vi "_emi_Version from VI tags.vi"(0 "vi reference":refnum<vi>, 11 "error in":errorcluster) -> (4 "vi Refnum out":refnum<vi>, 8 "Version Info":T1 {"Date" format="%<%y%m%d>T"}, 15 "error out":errorcluster)   [LabVIEW 2010]
doc: "Reads version information from a VI.\n\nIf it fails it does not transmitt error information on."
uses:
  emi_Version Info.ctl
  <vilib>/UserTags/UserTags.lvlib
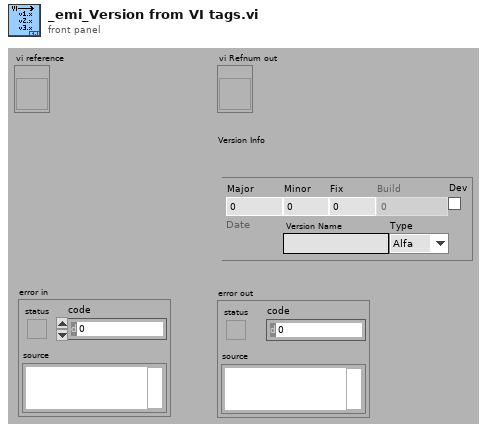
[diagram p1: front panel]
types:
  T1 = typedef "emi_Version Info.ctl" = cluster{"Name":string, "Major":i16, "Minor":i16, "Fix":i16, "Build":i32, "Type":enum16{"Alfa", "Beta", "Stable"}, "Dev":bool, "Version Name":string, "Date":timestamp}
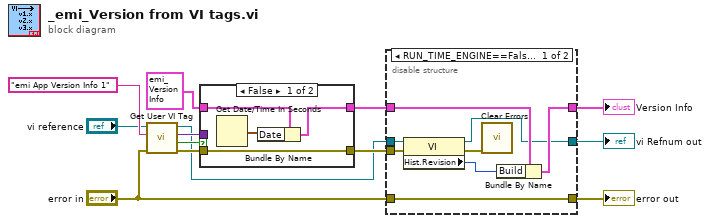
[diagram p0: block diagram]
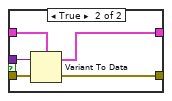
[diagram p3: hidden frame]
diagram:
  n1 = call <vilib>:"Get User VI Tag.vi"("error in (no error)"="error in", "Tag Name"="emi App Version Info 1", "VI Refnum"="vi reference") -> ("error out"=w7:errorcluster, "Was Tag Found?"=w8:bool, "Value"=w9:variant, "dup VI Refnum"=w5:refnum<vi>)  [unwired: 5 in]
  n2 = case shown="False" w8 {
    tunnel: [w15 w22] -> w10
    tunnel: w9 -> [_ w21]
    tunnel: w7 -> [w16 w20]
    tunnel: [w16 w19] -> w6
    tunnel: T1 {"Name"="NA", "Major"=0, "Minor"=0, "Fix"=0, "Build"=0, "Type"=enum."Alfa", "Dev"=TRUE, "Version Name"="", "Date"=timestamp(0 s since 1904-01-01)} ("Version Info") -> [w17 w18]
    frame False {
      n3 = Get Date/Time In Seconds() -> (seconds since 1Jan1904=w14:timestamp)
      n4 = Bundle By Name(cluster=w17, "Date"=w14) -> (w15:T1)
    }
    frame True {
      n5 = Variant To Data(error in=w20, Variant=w21, type=w18) -> (error out=w19:errorcluster, data=w22:T1)
    }
  }
  n6 = disable-structure shown="RUN_TIME_ENGINE==False" {
    disable-tunnel: [w30 w31] -> w11
    disable-tunnel: w10 -> [w29 w31]
    disable-tunnel: w6 -> [w27 _]
    disable-tunnel: w5 -> [w26 w33]
    disable-tunnel: [w23 w32] -> w3
    disable-tunnel: [w24 w33] -> w2
    disable-tunnel: "error in" -> [w23 w32]
    frame condition #0 (active) {
      n7 = property class="VI"(reference=w26, error in=w27) -> (reference out=w24:refnum<vi>, error out=w25:errorcluster, "Hist.Revision"=w28:u32)
      n8 = call <vilib>:"Clear Errors.vi"("error in (no error)"=w25) -> ()  [unwired: 6 in, 1 out]
      n9 = Bundle By Name(cluster=w29, "Build"=w28) -> (w30:T1)
    }
    frame condition #1 {
    }
  }
  "Version Info" <- w11
  "vi Refnum out" <- w2
  "error out" <- w3
